vi "half sub & full sub.vi"() -> ()   [LabVIEW 2025]
panel:
  in  "c":bool
  out "barrow 2":bool
  out "diff 2":bool
  in  "b":bool
  in  "a":bool
  out "barrow":bool
  out "diff":bool
  in  "a":bool
  in  "b":bool
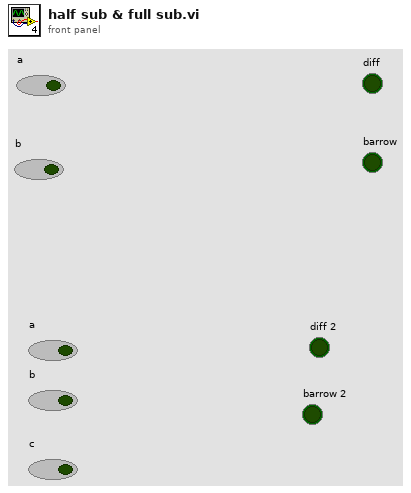
[diagram p1: front panel]
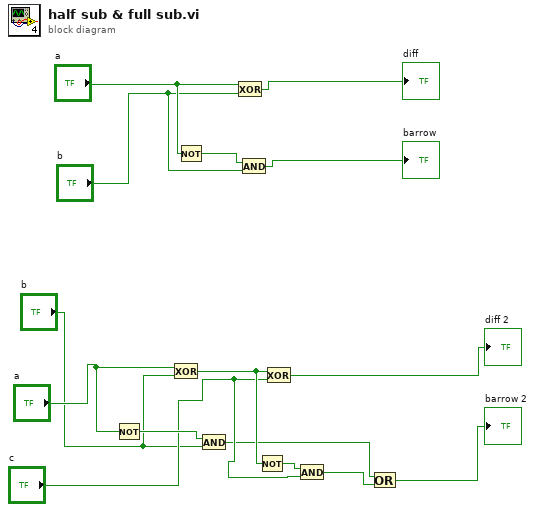
[diagram p0: block diagram]
diagram:
  n1 = Not(x="a") -> (.not. x?=w10:bool)
  n2 = Exclusive Or(1:"b", 2:"a") -> (0:w8:bool)
  n3 = Not(x="a") -> (.not. x?=w15:bool)
  n4 = And(x=w10, y="b") -> (x .and. y?=w6:bool)
  n5 = Exclusive Or(1:"b", 2:"a") -> (0:→"diff":bool)
  n6 = And(x=w15, y="b") -> (x .and. y?=→"barrow":bool)
  n7 = Not(x=w8) -> (.not. x?=w9:bool)
  n8 = Exclusive Or(1:"c", 2:w8) -> (0:→"diff 2":bool)
  n9 = And(x=w9, y="c") -> (x .and. y?=w5:bool)
  n10 = Or(x=w6, y=w5) -> (x .or. y?=→"barrow 2":bool)
